vi "Write Recurse.vi"(7 "Append Name (T)":bool=TRUE, 8 "Error In":errorcluster, 10 "Name":string, 11 "Variant":variant) -> (0 "Error Out":errorcluster, 2 "String":string)   [LabVIEW 2017, in "Configit.lvlib"]
uses:
  Configit.lvlib
  <vilib>/Waveform/DTblOps.llb/DTbl Empty Digital.vi
  <vilib>/Waveform/DWDTOps.llb/DWDT Empty Digital.vi
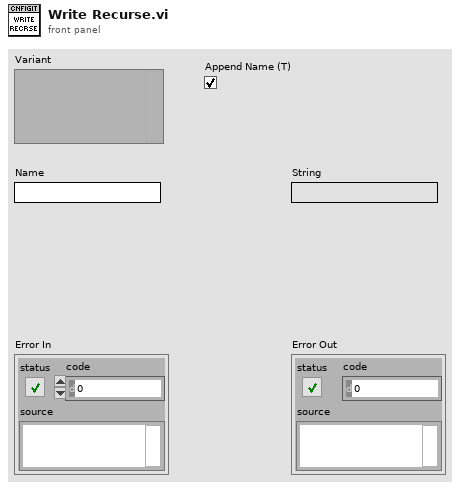
[diagram p1: front panel]
types:
  T1 = typedef "VariantType.lvlib/Type.ctl" = enum8{"Invalid Type", "Void", "I8", "I16", "I32", "I64", "U8", "U16", "U32", "U64", "Single Float", "Double Float", "Extended Float", "Single Complex", "Double Complex", "Extended Complex", "Enum U8", "Enum U16", "Enum U32", "Enum U64", "Single Float With Unit", "Double Float With Unit", "Extended Float With Unit", "Single Complex with Unit", "Double Complex with Unit", "Extended Complex with Unit", "Boolean", "String", "Path", "Picture", "Tag", "Array", "Cluster", "Variant", "LV Variant", "Waveform", "Timestamp", "Digital Waveform", "Digital Data", "ExpressData", "Refnum", "External Data", "VI", "Poly VI", "LabVIEW Class Instance", "Fixed Point"}
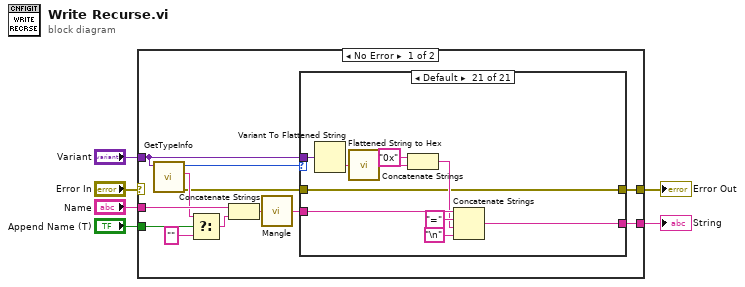
[diagram p0: block diagram]
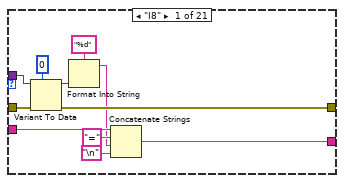
[diagram p2: hidden frame]
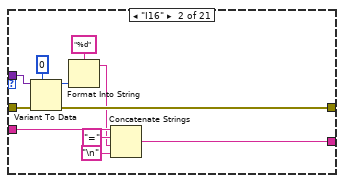
[diagram p3: hidden frame]
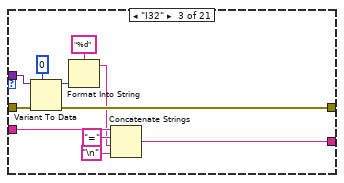
[diagram p4: hidden frame]
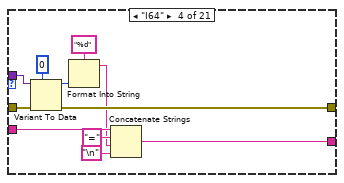
[diagram p5: hidden frame]
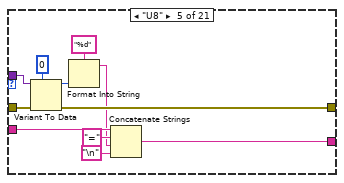
[diagram p6: hidden frame]
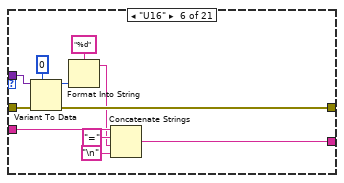
[diagram p7: hidden frame]
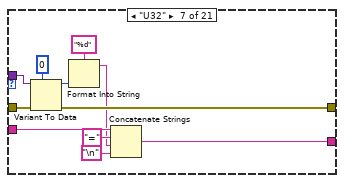
[diagram p8: hidden frame]
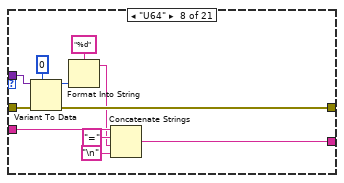
[diagram p9: hidden frame]
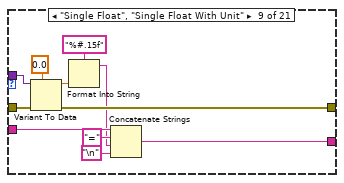
[diagram p10: hidden frame]
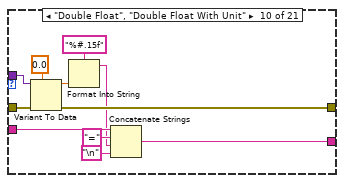
[diagram p11: hidden frame]
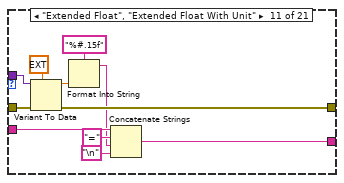
[diagram p12: hidden frame]
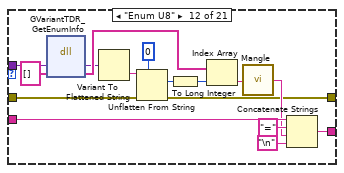
[diagram p13: hidden frame]
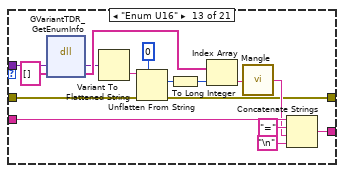
[diagram p14: hidden frame]
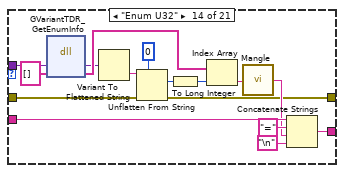
[diagram p15: hidden frame]
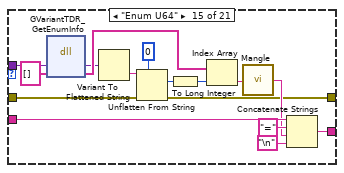
[diagram p16: hidden frame]
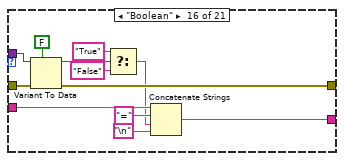
[diagram p17: hidden frame]
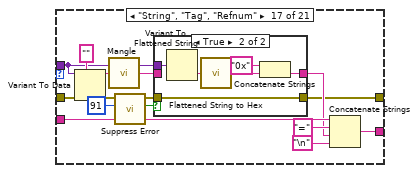
[diagram p18: hidden frame]
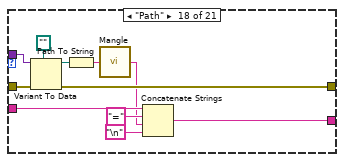
[diagram p20: hidden frame]
diagram:
  n1 = case shown="No Error" "Error In" {
    selector: "Error In" -> [_ w282]
    tunnel: "Variant" -> [w12 _]
    tunnel: "Name" -> [w18 _]
    tunnel: [w7 w282] -> w3
    tunnel: [w8 _] -> w2
    tunnel: "Append Name (T)" -> [w17 _]
    frame No Error {
      n2 = call "GetTypeInfo.vi"("Variant"=w12) -> ("Error Out"=w11:errorcluster, "Name"=w16:string, "Type Enum"=w13:T1)  [unwired: 7 in, 1 out]
      n3 = Select(t=w16, s=w17, f="") -> (s? t:f=w15:string)
      n4 = Concatenate Strings(w18, w15) -> (w10:string)
      n5 = call "Mangle.vi"("String In"=w10) -> ("String Out"=w9:string)
      n6 = case shown="Default" w13 {
        tunnel: w12 -> [w28 w39 w50 w61 w72 w83 w94 w105 w116 w127 w138 w141 w157 w173 w189 w214 w216 w248 w252 w264 w281]
        tunnel: w11 -> [w29 w40 w51 w62 w73 w84 w95 w106 w117 w128 w139 w148 w164 w180 w196 w215 w230 w249 w254 w265 w272]
        tunnel: w9 -> [w24 w35 w46 w57 w68 w79 w90 w101 w112 w123 w134 w153 w169 w185 w201 w211 w227 w245 w253 w260 w278]
        tunnel: [w23 w34 w45 w56 w67 w78 w89 w100 w111 w122 w133 w152 w168 w184 w200 w210 w226 w244 w250 w255 w276] -> w8
        tunnel: [w22 w33 w44 w55 w66 w77 w88 w99 w110 w121 w132 w142 w158 w174 w190 w209 w217 w243 w251 w256 w272] -> w7
        frame "I8" {
          n7 = Variant To Data(error in=w29, type=i8 0, Variant=w28) -> (data=w21:i8, error out=w22:errorcluster)
          n8 = Format Into String(format string="%d", w21) -> (resulting string=w19:string)  [unwired: 2 in, 1 out]
          n9 = Concatenate Strings(w24, "=" ("string"), w19, "\n") -> (w23:string)
        }
        frame "I16" {
          n10 = Variant To Data(error in=w40, type=i16 0, Variant=w39) -> (data=w32:i16, error out=w33:errorcluster)
          n11 = Format Into String(format string="%d", w32) -> (resulting string=w30:string)  [unwired: 2 in, 1 out]
          n12 = Concatenate Strings(w35, "=" ("string"), w30, "\n") -> (w34:string)
        }
        frame "I32" {
          n13 = Variant To Data(error in=w51, type=0, Variant=w50) -> (data=w43:i32, error out=w44:errorcluster)
          n14 = Format Into String(format string="%d", w43) -> (resulting string=w41:string)  [unwired: 2 in, 1 out]
          n15 = Concatenate Strings(w46, "=" ("string"), w41, "\n") -> (w45:string)
        }
        frame "I64" {
          n16 = Variant To Data(error in=w62, type=i64 0, Variant=w61) -> (data=w54:i64, error out=w55:errorcluster)
          n17 = Format Into String(format string="%d", w54) -> (resulting string=w52:string)  [unwired: 2 in, 1 out]
          n18 = Concatenate Strings(w57, "=" ("string"), w52, "\n") -> (w56:string)
        }
        frame "U8" {
          n19 = Variant To Data(error in=w73, type=u8 0, Variant=w72) -> (data=w65:u8, error out=w66:errorcluster)
          n20 = Format Into String(format string="%d", w65) -> (resulting string=w63:string)  [unwired: 2 in, 1 out]
          n21 = Concatenate Strings(w68, "=" ("string"), w63, "\n") -> (w67:string)
        }
        frame "U16" {
          n22 = Variant To Data(error in=w84, type=u16 0, Variant=w83) -> (data=w76:u16, error out=w77:errorcluster)
          n23 = Format Into String(format string="%d", w76) -> (resulting string=w74:string)  [unwired: 2 in, 1 out]
          n24 = Concatenate Strings(w79, "=" ("string"), w74, "\n") -> (w78:string)
        }
        frame "U32" {
          n25 = Variant To Data(error in=w95, type=u32 0, Variant=w94) -> (data=w87:u32, error out=w88:errorcluster)
          n26 = Format Into String(format string="%d", w87) -> (resulting string=w85:string)  [unwired: 2 in, 1 out]
          n27 = Concatenate Strings(w90, "=" ("string"), w85, "\n") -> (w89:string)
        }
        frame "U64" {
          n28 = Variant To Data(error in=w106, type=u64 0, Variant=w105) -> (data=w98:u64, error out=w99:errorcluster)
          n29 = Format Into String(format string="%d", w98) -> (resulting string=w96:string)  [unwired: 2 in, 1 out]
          n30 = Concatenate Strings(w101, "=" ("string"), w96, "\n") -> (w100:string)
        }
        frame "Single Float", "Single Float With Unit" {
          n31 = Variant To Data(error in=w117, type=sgl 0.0, Variant=w116) -> (data=w109:sgl, error out=w110:errorcluster)
          n32 = Format Into String(format string="%#.15f", w109) -> (resulting string=w107:string)  [unwired: 2 in, 1 out]
          n33 = Concatenate Strings(w112, "=" ("string"), w107, "\n") -> (w111:string)
        }
        frame "Double Float", "Double Float With Unit" {
          n34 = Variant To Data(error in=w128, type=0.0, Variant=w127) -> (data=w120:dbl, error out=w121:errorcluster)
          n35 = Format Into String(format string="%#.15f", w120) -> (resulting string=w118:string)  [unwired: 2 in, 1 out]
          n36 = Concatenate Strings(w123, "=" ("string"), w118, "\n") -> (w122:string)
        }
        frame "Extended Float", "Extended Float With Unit" {
          n37 = Variant To Data(error in=w139, type=ext 0.0, Variant=w138) -> (data=w131:ext, error out=w132:errorcluster)
          n38 = Format Into String(format string="%#.15f", w131) -> (resulting string=w129:string)  [unwired: 2 in, 1 out]
          n39 = Concatenate Strings(w134, "=" ("string"), w129, "\n") -> (w133:string)
        }
        frame "Enum U8" {
          n40 = dll-call lib="LabVIEW" fn="GVariantTDR_GetEnumInfo"("lvVar"=w141, "enumNames"=string[] []) -> ("lvVar"=w140:variant, "enumNames"=w143:string[])  [unwired: 4 in, 2 out]
          n41 = Variant To Flattened String(Variant=w140) -> (data string=w147:string)  [unwired: 1 out]
          n42 = Unflatten From String(type=u8 0, binary string=w147, error in (no error)=w148) -> (value=w149:u8, error out=w142:errorcluster)  [unwired: 2 in, 1 out]
          n43 = To Long Integer(number=w149) -> (32bit integer=w146:i32)
          n44 = Index Array(array=w143, index=w146) -> (element=w145:string)
          n45 = call "Mangle.vi"("String In"=w145) -> ("String Out"=w144:string)
          n46 = Concatenate Strings(w153, "=" ("string"), w144, "\n") -> (w152:string)
        }
        frame "Enum U16" {
          n47 = dll-call lib="LabVIEW" fn="GVariantTDR_GetEnumInfo"("lvVar"=w157, "enumNames"=string[] []) -> ("lvVar"=w156:variant, "enumNames"=w159:string[])  [unwired: 4 in, 2 out]
          n48 = Variant To Flattened String(Variant=w156) -> (data string=w163:string)  [unwired: 1 out]
          n49 = Unflatten From String(type=u16 0, binary string=w163, error in (no error)=w164) -> (value=w165:u16, error out=w158:errorcluster)  [unwired: 2 in, 1 out]
          n50 = To Long Integer(number=w165) -> (32bit integer=w162:i32)
          n51 = Index Array(array=w159, index=w162) -> (element=w161:string)
          n52 = call "Mangle.vi"("String In"=w161) -> ("String Out"=w160:string)
          n53 = Concatenate Strings(w169, "=" ("string"), w160, "\n") -> (w168:string)
        }
        frame "Enum U32" {
          n54 = dll-call lib="LabVIEW" fn="GVariantTDR_GetEnumInfo"("lvVar"=w173, "enumNames"=string[] []) -> ("lvVar"=w172:variant, "enumNames"=w175:string[])  [unwired: 4 in, 2 out]
          n55 = Variant To Flattened String(Variant=w172) -> (data string=w179:string)  [unwired: 1 out]
          n56 = Unflatten From String(type=u32 0, binary string=w179, error in (no error)=w180) -> (value=w181:u32, error out=w174:errorcluster)  [unwired: 2 in, 1 out]
          n57 = To Long Integer(number=w181) -> (32bit integer=w178:i32)
          n58 = Index Array(array=w175, index=w178) -> (element=w177:string)
          n59 = call "Mangle.vi"("String In"=w177) -> ("String Out"=w176:string)
          n60 = Concatenate Strings(w185, "=" ("string"), w176, "\n") -> (w184:string)
        }
        frame "Enum U64" {
          n61 = dll-call lib="LabVIEW" fn="GVariantTDR_GetEnumInfo"("lvVar"=w189, "enumNames"=string[] []) -> ("lvVar"=w188:variant, "enumNames"=w191:string[])  [unwired: 4 in, 2 out]
          n62 = Variant To Flattened String(Variant=w188) -> (data string=w195:string)  [unwired: 1 out]
          n63 = Unflatten From String(type=u64 0, binary string=w195, error in (no error)=w196) -> (value=w197:u64, error out=w190:errorcluster)  [unwired: 2 in, 1 out]
          n64 = To Long Integer(number=w197) -> (32bit integer=w194:i32)
          n65 = Index Array(array=w191, index=w194) -> (element=w193:string)
          n66 = call "Mangle.vi"("String In"=w193) -> ("String Out"=w192:string)
          n67 = Concatenate Strings(w201, "=" ("string"), w192, "\n") -> (w200:string)
        }
        frame "Boolean" {
          n68 = Variant To Data(error in=w215, type=FALSE, Variant=w214) -> (data=w207:bool, error out=w209:errorcluster)
          n69 = Select(t="True", s=w207, f="False") -> (s? t:f=w206:string)
          n70 = Concatenate Strings(w211, "=" ("string"), w206, "\n") -> (w210:string)
        }
        frame "String", "Tag", "Refnum" {
          n71 = Variant To Data(error in=w230, type="" ("f"), Variant=w216) -> (data=w224:string, error out=w223:errorcluster)
          n72 = call "Mangle.vi"("String In"=w224) -> ("String Out"=w219:string)
          n73 = call "Suppress Error.vi"("Error Code"=91, "Error In"=w223) -> ("Error Supressed?"=w221:bool, "Error Out"=w218:errorcluster)  [unwired: 4 in]
          n74 = case shown="True" w221 {
            tunnel: [w232 w235] -> w220
            tunnel: w219 -> [w232 _]
            tunnel: w218 -> [w231 w233]
            tunnel: [w231 w233] -> w217
            tunnel: w216 -> [_ w234]
            frame False {
            }
            frame True {
              n75 = Variant To Flattened String(Variant=w234) -> (data string=w237:string)  [unwired: 1 out]
              n76 = call "Flattened String to Hex.vi"("Flattened String"=w237) -> ("Hex"=w236:string)
              n77 = Concatenate Strings("0x", w236) -> (w235:string)
            }
          }
          n78 = Concatenate Strings(w227, "=" ("string"), w220, "\n") -> (w226:string)
        }
        frame "Path" {
          n79 = Variant To Data(error in=w249, type=path "", Variant=w248) -> (data=w240:path, error out=w243:errorcluster)
          n80 = Path To String(path=w240) -> (string=w239:string)
          n81 = call "Mangle.vi"("String In"=w239) -> ("String Out"=w242:string)
          n82 = Concatenate Strings(w245, "=" ("string"), w242, "\n") -> (w244:string)
        }
        frame "Array" {
          n83 = call "Write Array.vi"("Error In"=w254, "Name"=w253, "Variant"=w252) -> ("Error Out"=w251:errorcluster, "String"=w250:string)  [unwired: 7 in]
        }
        frame "Cluster" {
          n84 = Variant To Data(error in=w265, type=variant[] [], Variant=w264) -> (data=w262:variant[], error out=w263:errorcluster)
          n85 = Concatenate Strings(w260, "." ("string")) -> (w259:string)
          n86 = for {
            tunnel: w263 -> [w271]
            tunnel: w262 -> [w270] mode=indexing
            tunnel: w259 -> [w269]
            tunnel: [w268] -> w257 mode=indexing
            workers-P: _ -> [_]
            tunnel: [w267] -> w258 mode=indexing
            n87 = call "Write Recurse.vi"("Error In"=w271, "Name"=w269, "Variant"=w270) -> ("Error Out"=w268:errorcluster, "String"=w267:string)  [unwired: 7 in]
          }
          n88 = Concatenate Strings(w258) -> (w255:string)
          n89 = Merge Errors(w257) -> (w256:errorcluster)
        }
        frame Default {
          n90 = Variant To Flattened String(Variant=w281) -> (data string=w275:string)  [unwired: 1 out]
          n91 = call "Flattened String to Hex.vi"("Flattened String"=w275) -> ("Hex"=w274:string)
          n92 = Concatenate Strings("0x", w274) -> (w273:string)
          n93 = Concatenate Strings(w278, "=" ("string"), w273, "\n") -> (w276:string)
        }
      }
    }
    frame Error {
    }
  }
  "Error Out" <- w3
  "String" <- w2
